vi "Set Macro by Name.vi"(8 "error in (no error)":errorcluster, 9 "TriggerAction Q.lvclass":refnum<class "TriggerAction Q.lvclass">, 10 "Macro Name":string, 11 "Motions in":refnum<class "Motions.lvclass">) -> (0 "error out":errorcluster, 3 "Motions out":refnum<class "Motions.lvclass">)   [LabVIEW 2016, in "Hardware.lvlib" / "Motions.lvlib" / "Motions.lvclass"]
uses:
  <userlib>/Common Components/Hardware/Abstract System/Motions/Motions/Motions.lvclass
  <userlib>/Common Components/TriggerAction Q/TriggerAction Q/TriggerAction Q.lvclass
  <userlib>/Common Components/Hardware/Abstract System/Motions/Motions/Motions.lvclass/Motions.ctl
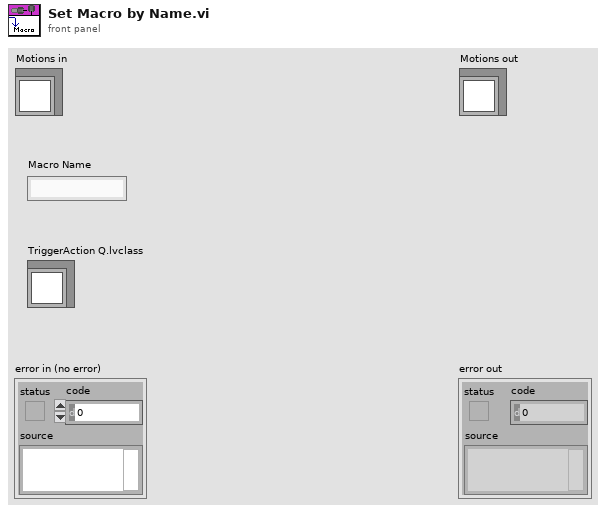
[diagram p1: front panel]
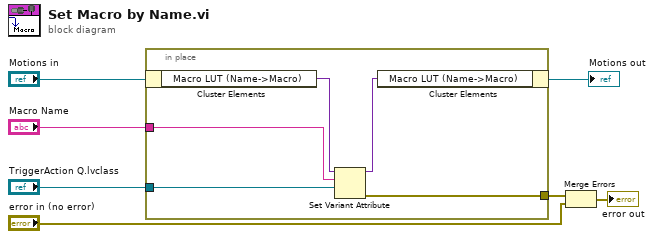
[diagram p0: block diagram]
diagram:
  n1 = in-place {
    in-place-border: "Macro Name" -> [w10]
    in-place-border: "TriggerAction Q.lvclass" -> [w9]
    in-place-border: [w8] -> w2
    n2 = in-place-cluster #1("Motions in") -> ("Macro LUT (Name->Macro)"=w12:variant)
    n3 = Set Variant Attribute(Variant=w12, name=w10, value=w9) -> (Variant out=w11:variant, error out=w8:errorcluster)  [unwired: 1 in, 1 out]
    n4 = in-place-cluster #1("Macro LUT (Name->Macro)"=w11) -> (→"Motions out":refnum<class "Motions.lvclass">)
  }
  n5 = Merge Errors(w2, "error in (no error)") -> (→"error out":errorcluster)
